vi "Abs.vi"(0 "controller in":refnum<k24>, 11 "error in (no error)":errorcluster) -> (4 "controller out":refnum<k24>, 15 "error out":errorcluster)   [LabVIEW 2019]
uses:
  C:/Users/patrick/Documents/GitHub/Aerotech-Delay-Line/lvsrc/Aerotech-Ensemble-LabVIEW/2010-5.6/Bin/Aerotech.Ensemble.dll
  Bin/Aerotech.Ensemble.dll
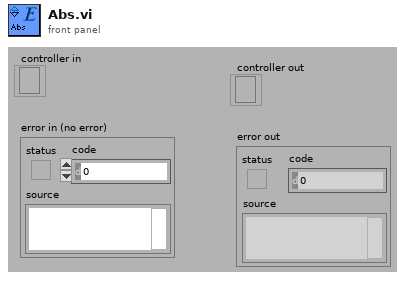
[diagram p1: front panel]
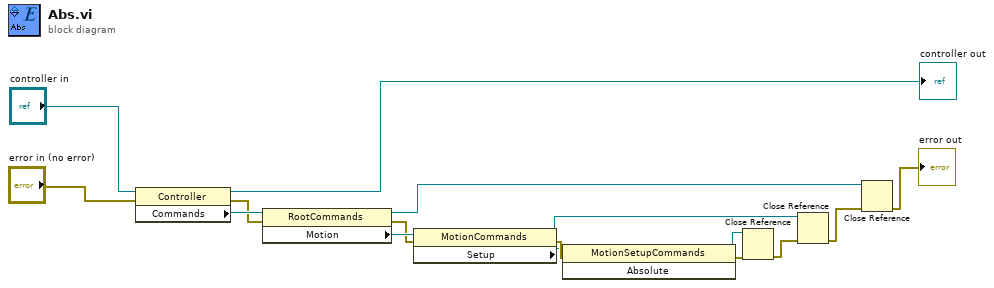
[diagram p0: block diagram]
diagram:
  n1 = property class="Controller"(reference="controller in", error in="error in (no error)") -> (reference out=→"controller out":refnum<k24>, error out=w12:errorcluster, "Commands"=w13:refnum<k24>)
  n2 = property class="RootCommands"(reference=w13, error in=w12) -> (reference out=w9:refnum<k24>, error out=w7:errorcluster, "Motion"=w8:refnum<k24>)
  n3 = property class="MotionCommands"(reference=w8, error in=w7) -> (reference out=w6:refnum<k24>, error out=w5:errorcluster, "Setup"=w4:refnum<k24>)
  n4 = invoke class="MotionSetupCommands" method="Absolute"(reference=w4, error in=w5) -> (reference out=w2:refnum<k24>, error out=w3:errorcluster)  [unwired: 1 in, 1 out]
  n5 = Close Reference(reference=w2, error in (no error)=w3) -> (error out=w1:errorcluster)
  n6 = Close Reference(reference=w6, error in (no error)=w1) -> (error out=w10:errorcluster)
  n7 = Close Reference(reference=w9, error in (no error)=w10) -> (error out=→"error out":errorcluster)
